vi "初始化检查与创建.vi"(6 "模式(读取)":enum16{"读取", "写入"}(ring), 7 "配置文件 i":T1 {"定时配置-自动导出"."定时配置-自动导出"."间隔" min=1; "定时配置-累积分段"."间隔" min=1}, 8 "error in (no error)":errorcluster caption="错误输入（无错误）", 11 "配置文件路径":path) -> (0 "error out":errorcluster caption="错误输出", 3 "配置文件 o":T1 {"定时配置-自动导出"."定时配置-自动导出"."间隔" min=1; "定时配置-累积分段"."间隔" min=1})   [LabVIEW 2017]
uses:
  a3565fc4-ee2f-4113-b32d-f6e48cc88c0d.vi
  582f122c-475a-4877-9f1d-e028bce6f79a.vi
  9617da62-d855-45df-82b1-57c8dcb712c4.vi
  c94f7198-3dea-4324-b842-01edaf5fdd37.vi
  494809bb-0510-4db4-aacf-66d689d66c07.vi
  <vilib>/Utility/config.llb/Read Key (Boolean).vi
  <vilib>/Utility/config.llb/Write Key (Boolean).vi
  <vilib>/Utility/config.llb/Read Key (String).vi
  <vilib>/Utility/config.llb/Write Key (String).vi
  <vilib>/Utility/config.llb/Read Key (U32).vi
  <vilib>/Utility/config.llb/Write Key (U32).vi
  <vilib>/Utility/config.llb/Write Key (I32).vi
  <vilib>/Utility/config.llb/NI_LVConfig.lvlib
panel:
  in  "键-导出定时配置段":T4
  in  "键-累积定时配置段":T5
  in  "键-串口配置段":T6
  in  "键-杂项段":T7
  in  "段":T8
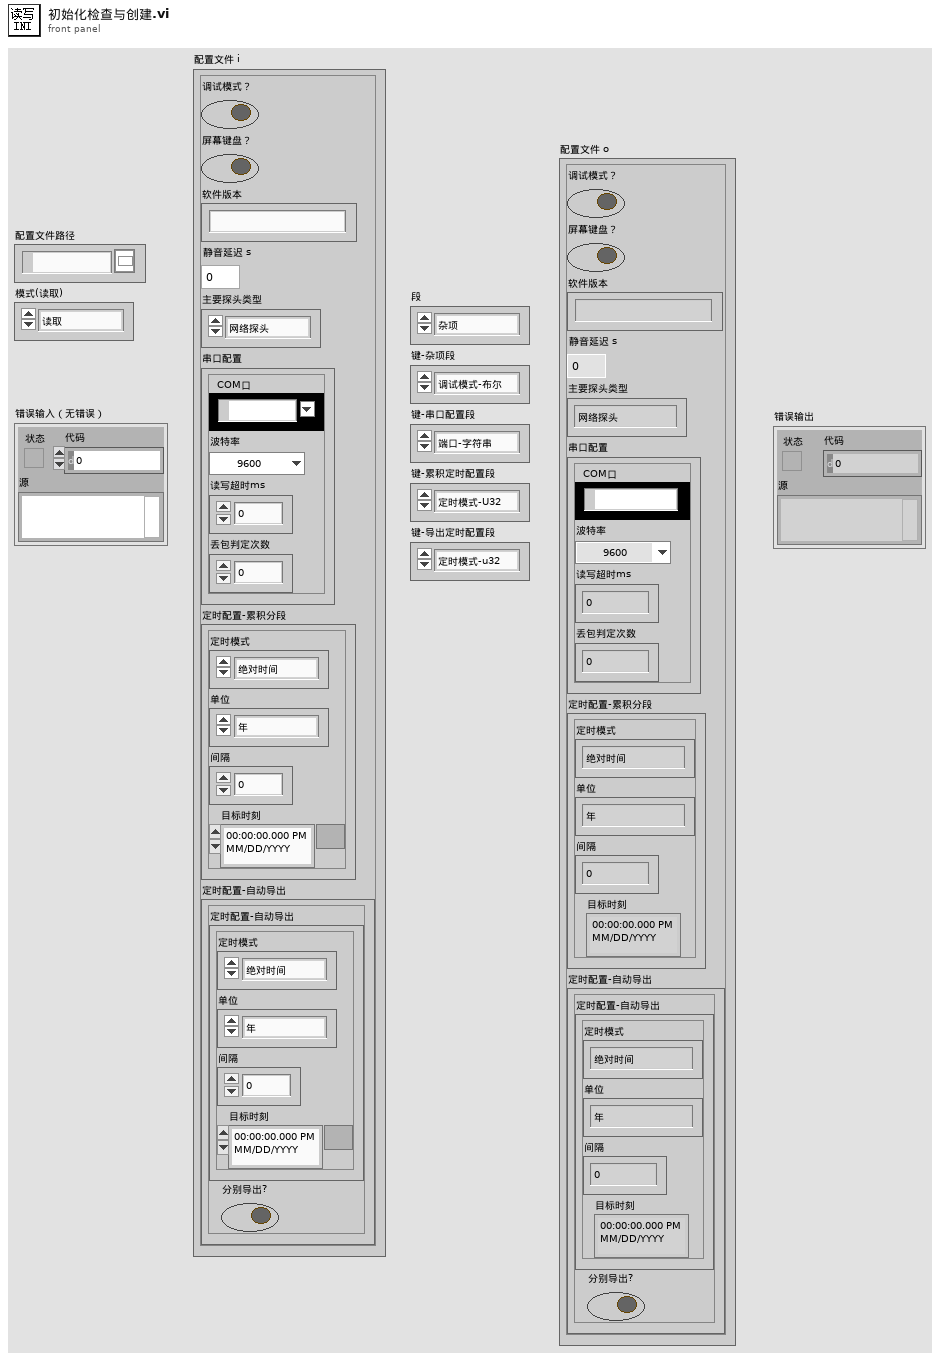
[diagram p1: front panel]
types:
  T1 = typedef "簇-配置文件内容.ctl" = cluster{"调试模式？":bool, "屏幕键盘？":bool, "软件版本":string, "静音延迟 s":u16, "主要探头类型":T2, "串口配置":cluster{"COM口":refnum<visa-resource-name>, "波特率":enum16{"9600", "19200"}, "读写超时ms":i16, "丢包判定次数":i16}, "定时配置-累积分段":T3, "定时配置-自动导出":cluster{"定时配置-自动导出":T3, "分别导出?":bool}}
  T2 = typedef "枚举-主要探头类型.ctl" = enum16{"网络探头", "串口探头"}
  T3 = typedef "簇-定时配置.ctl" = cluster{"定时模式":enum16{"绝对时间", "相对时间"}, "单位":enum16{"年", "月", "日", "时", "分"}, "间隔":u8, "目标时刻":timestamp}
  T4 = typedef "枚举-键-导出定时配置段.ctl" = enum16{"定时模式-u32", "单位-u32", "间隔-u32", "目标时刻-字符串", "分别导出-布尔"}
  T5 = typedef "枚举-键-累积定时配置段.ctl" = enum16{"定时模式-U32", "单位-U32", "间隔-U32", "目标时刻-字符串"}
  T6 = typedef "枚举-键-串口配置段.ctl" = enum16{"端口-字符串", "波特率-U32", "读写超时ms-U32", "丢包判定次数-U32"}
  T7 = typedef "枚举-键-杂项段.ctl" = enum16{"调试模式-布尔", "屏幕键盘-布尔", "软件版本-字符串", "静音延迟-U32", "主要探头类型-U32"}
  T8 = typedef "枚举-段.ctl" = enum16{"杂项", "串口配置", "累积分段定时", "自动导出定时"}
  T9 = cluster{"COM口":refnum<visa-resource-name>, "波特率":enum16{"9600", "19200"}, "读写超时ms":i16, "丢包判定次数":i16}
  T10 = typedef "NI_LVConfig.lvlib/Config Data RefNum.ctl" = refnum<k1>
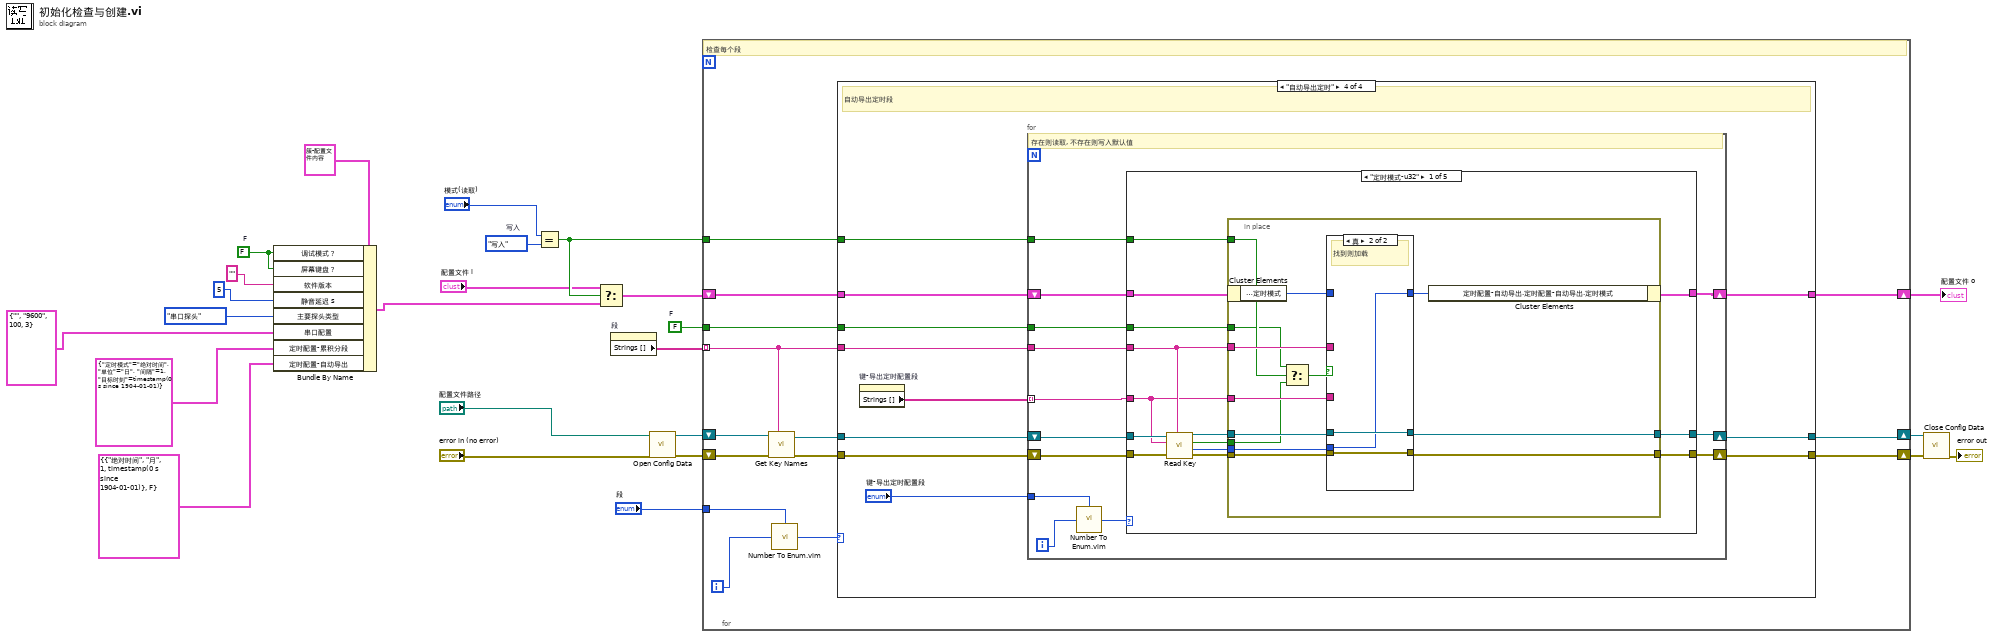
[diagram p0: block diagram]
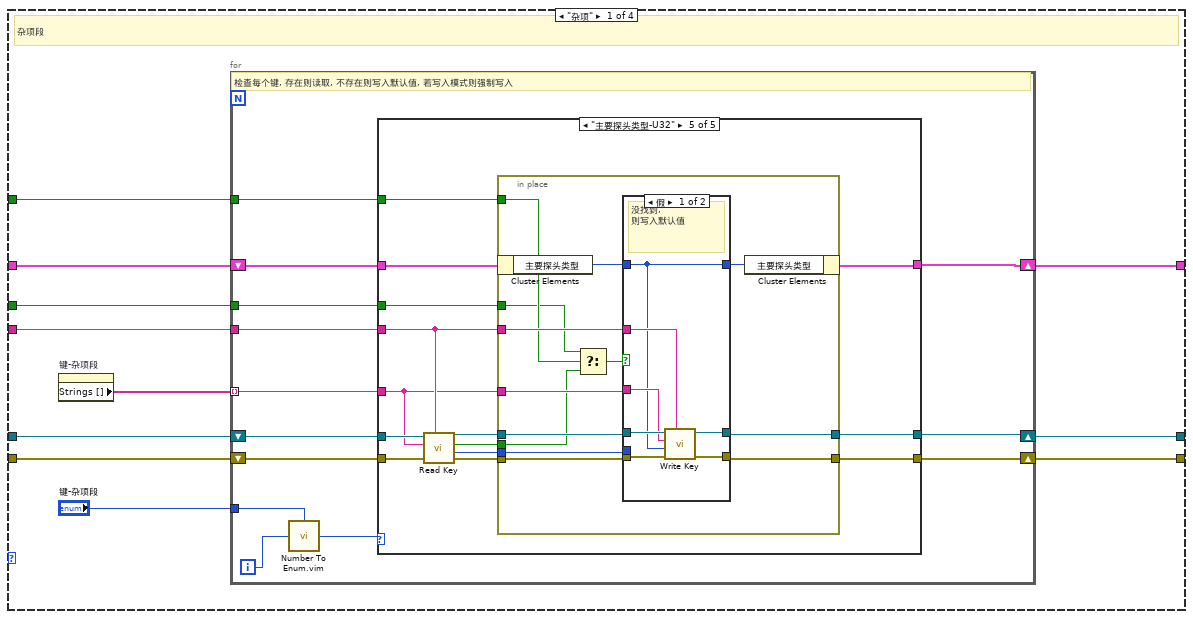
[diagram p2: hidden frame]
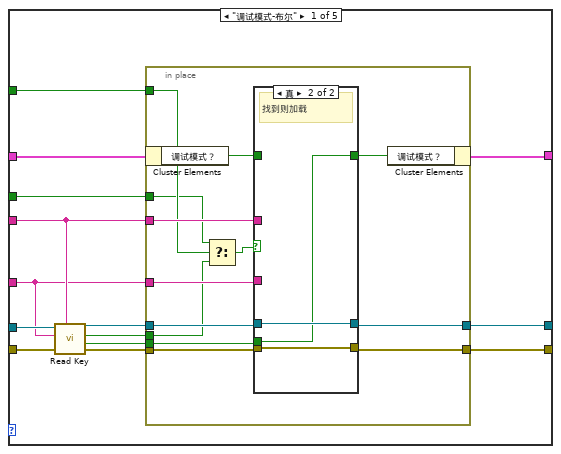
[diagram p3: hidden frame]
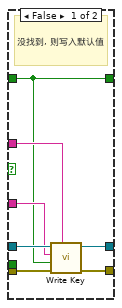
[diagram p4: hidden frame]
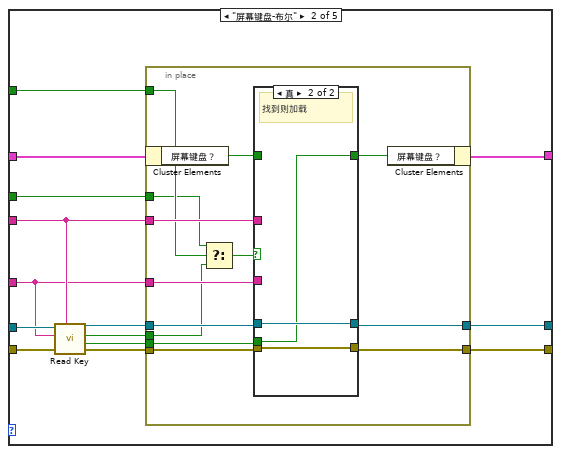
[diagram p5: hidden frame]
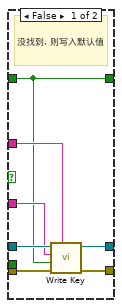
[diagram p6: hidden frame]
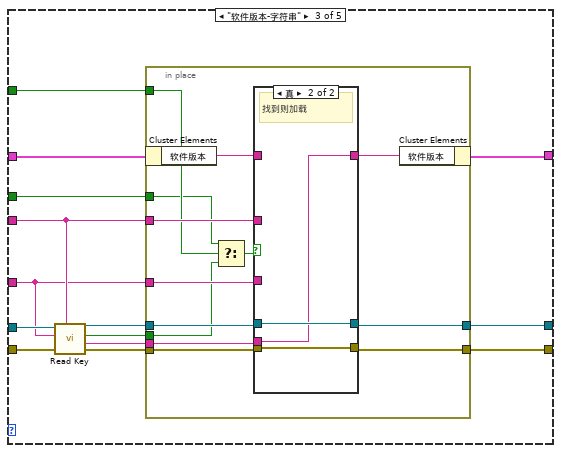
[diagram p7: hidden frame]
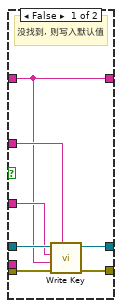
[diagram p8: hidden frame]
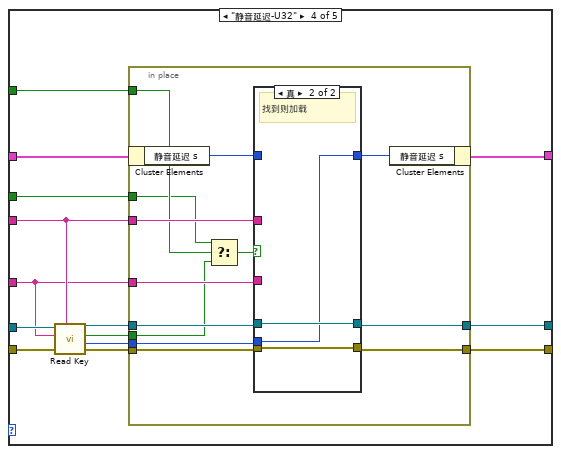
[diagram p9: hidden frame]
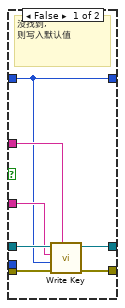
[diagram p10: hidden frame]
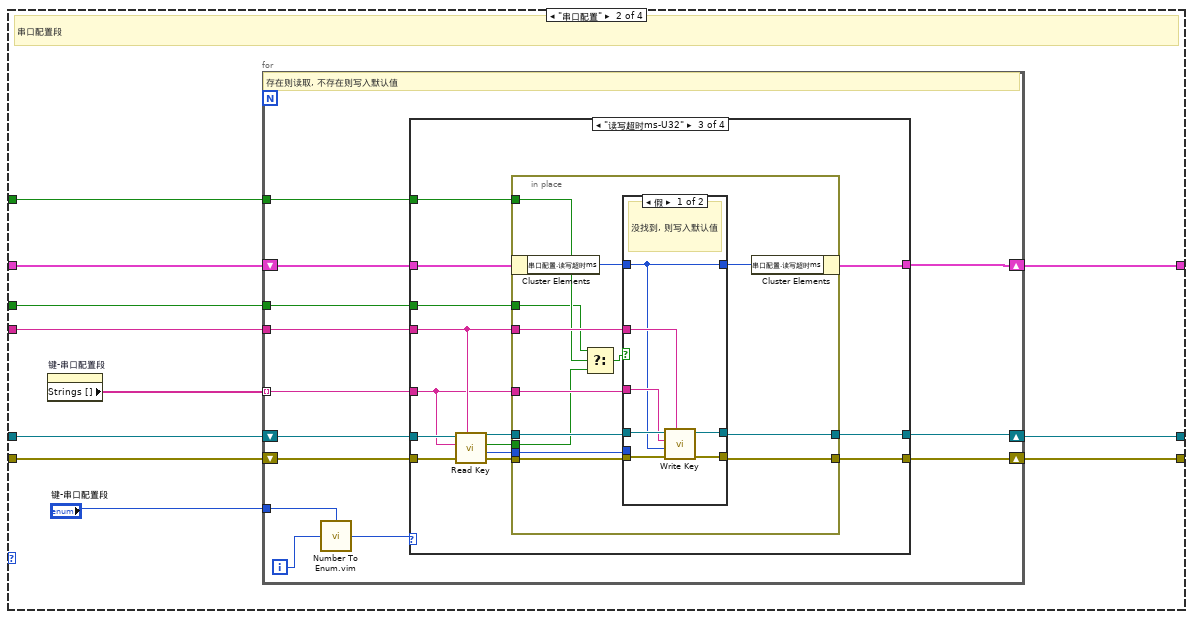
[diagram p12: hidden frame]
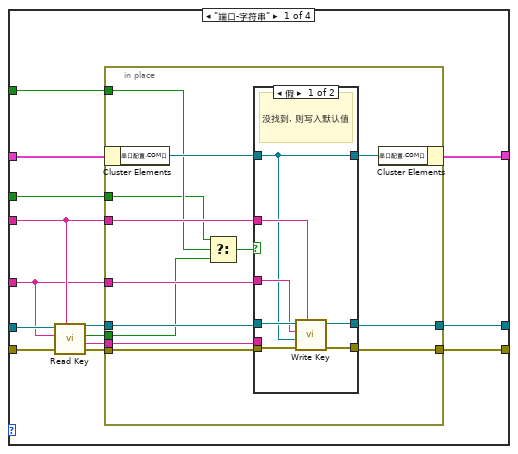
[diagram p13: hidden frame]
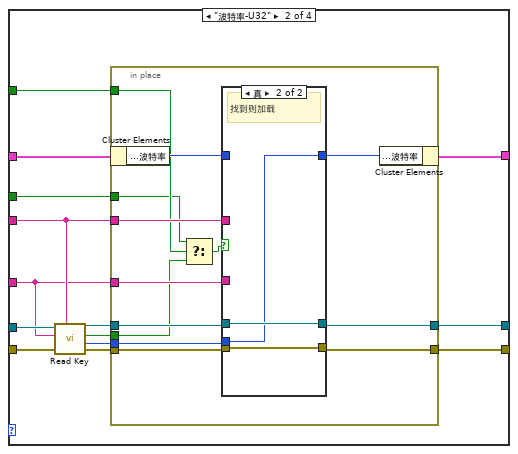
[diagram p15: hidden frame]
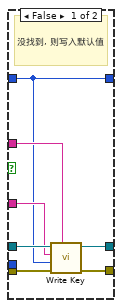
[diagram p16: hidden frame]
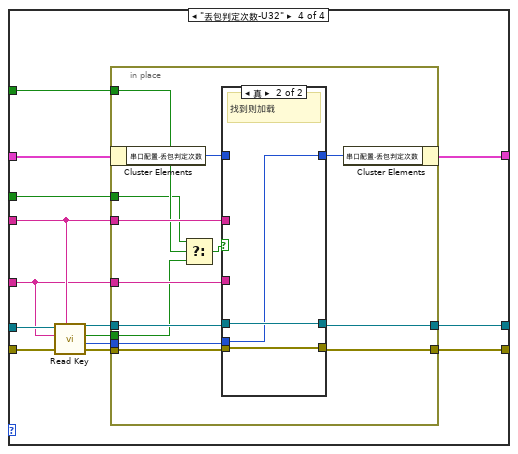
[diagram p18: hidden frame]
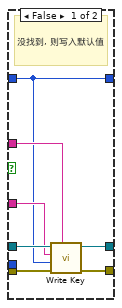
[diagram p19: hidden frame]
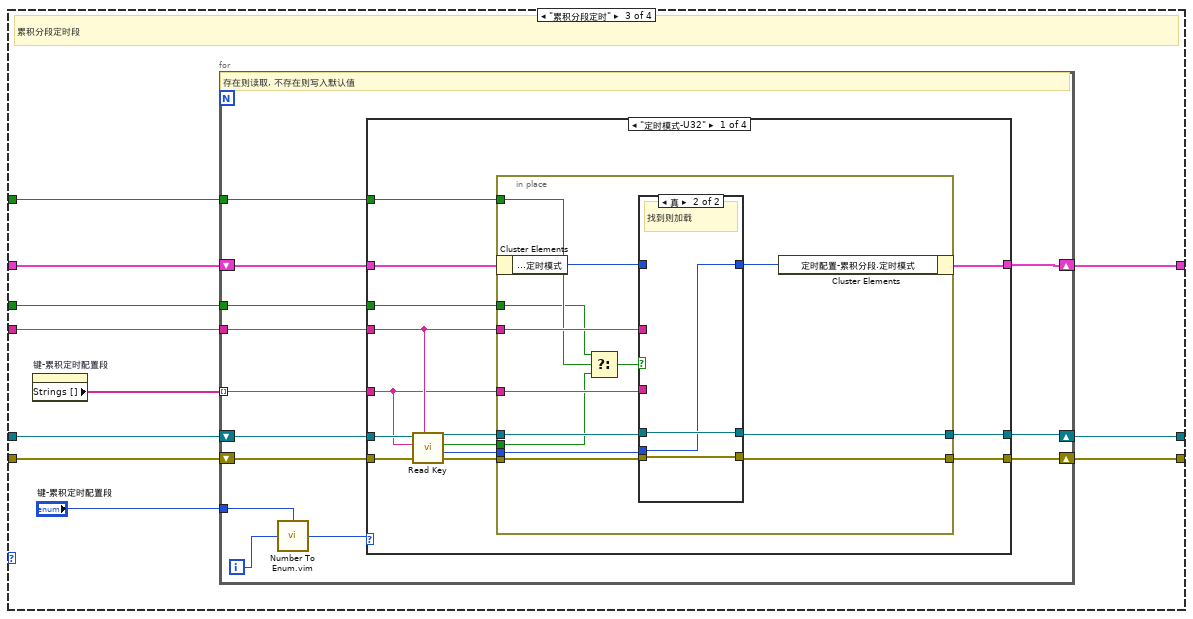
[diagram p20: hidden frame]
diagram:
  w5 = FALSE  # F
  w13 = FALSE  # F
  w14 = enum16{"读取", "写入"}."写入"  # 写入
  n1 = Bundle By Name(cluster=T1 {"调试模式？"=FALSE, "屏幕键盘？"=FALSE, "软件版本"="", "静音延迟 s"=0, "主要探头类型"=enum."网络探头", "串口配置"={"COM口"="", "波特率"=enum."9600", "读写超时ms"=0, "丢包判定次数"=0}, "定时配置-累积分段"={"定时模式"=enum."绝对时间", "单位"=enum."年", "间隔"=0, "目标时刻"=timestamp(0 s since 1904-01-01)}, "定时配置-自动导出"={"定时配置-自动导出"={"定时模式"=enum."绝对时间", "单位"=enum."年", "间隔"=0, "目标时刻"=timestamp(0 s since 1904-01-01)}, "分别导出?"=FALSE}} ("配置文件 i"), "调试模式？"=w5, "屏幕键盘？"=w5, "软件版本"="", "静音延迟 s"=u16 5, "主要探头类型"=枚举-主要探头类型."串口探头", "串口配置"=T9 {"COM口"="", "波特率"=enum."9600", "读写超时ms"=100, "丢包判定次数"=3}, "定时配置-累积分段"=T3 {"定时模式"=enum."绝对时间", "单位"=enum."日", "间隔"=1, "目标时刻"=timestamp(0 s since 1904-01-01)}, "定时配置-自动导出"=cluster{"定时配置-自动导出":T3, "分别导出?":bool} {"定时配置-自动导出"={"定时模式"=enum."绝对时间", "单位"=enum."月", "间隔"=1, "目标时刻"=timestamp(0 s since 1904-01-01)}, "分别导出?"=FALSE}) -> (w3:T1)
  n2 = Equal?(x="模式(读取)", y=w14) -> (x = y?=w12:bool)
  n3 = Select(t="配置文件 i", s=w12, f=w3) -> (s? t:f=w10:T1)
  n4 = property on="段" class="Enum (严格)"() -> ("Strings []"=w23:string[])  [unwired: 2 in, 2 out]
  n5 = call <vilib>:"Open Config Data.vi"("error in (no error)"="error in (no error)", "configuration file path"="配置文件路径") -> ("error out"=w17:errorcluster, "refnum"=w24:T10)  [unwired: 7 in, 1 out]
  n6 = for {
    tunnel: w23 -> [w34] mode=indexing
    shift-right: [w28] -> w22
    shift-left: w10 -> [w33]
    shift-right: [w29] -> w19
    shift-left: w24 -> [w39]
    shift-right: [w30] -> w20
    shift-left: w17 -> [w31]
    tunnel: "段" -> [w36]
    tunnel: w12 -> [w27]
    tunnel: w13 -> [w26]
    i -> [w37]
    # "检查每个段"
    n7 = call <vilib>:"Get Key Names.vi"("section"=w34, "error in (no error)"=w31, "refnum"=w39) -> ("error out"=w32:errorcluster, "refnum out"=w38:T10)  [unwired: 5 in, 2 out]
    n8 = call "Number To Enum.vim"("number"=w37, "enum type"=w36) -> ("number as enum"=w35:T8)
    n9 = case shown="\"自动导出定时\"" w35 {
      tunnel: w38 -> [w49 w259 w431 w606]
      tunnel: w34 -> [w48 w258 w430 w605]
      tunnel: w33 -> [w47 w257 w429 w604]
      tunnel: w32 -> [w45 w256 w428 w603]
      tunnel: [w44 w255 w427 w602] -> w30
      tunnel: [w43 w254 w426 w601] -> w29
      tunnel: [w42 w251 w423 w598] -> w28
      tunnel: w27 -> [w41 w250 w421 w597]
      tunnel: w26 -> [w40 w249 w422 w596]
      frame "杂项" {
        # "杂项段"
        n10 = property on="键-杂项段" class="Enum (严格)"() -> ("Strings []"=w50:string[])  [unwired: 2 in, 2 out]
        n11 = for {
          tunnel: w50 -> [w61] mode=indexing
          tunnel: w48 -> [w62]
          shift-right: [w53] -> w42
          shift-left: w47 -> [w57]
          tunnel: "键-杂项段" -> [w59]
          shift-right: [w54] -> w43
          shift-left: w49 -> [w63]
          shift-right: [w55] -> w44
          shift-left: w45 -> [w56]
          tunnel: w41 -> [w52]
          tunnel: w40 -> [w51]
          i -> [w60]
          # "检查每个键, 存在则读取, 不存在则写入默认值, 若写入模式则强制写入"
          n12 = call "Number To Enum.vim"("number"=w60, "enum type"=w59) -> ("number as enum"=w58:T7)
          n13 = case shown="\"主要探头类型-U32\"" w58 {
            tunnel: w63 -> [w77 w114 w151 w188 w225]
            tunnel: w62 -> [w74 w111 w148 w185 w222]
            tunnel: w61 -> [w73 w110 w147 w184 w221]
            tunnel: w57 -> [w67 w104 w141 w178 w215]
            tunnel: w56 -> [w71 w108 w145 w182 w219]
            tunnel: [w70 w107 w144 w181 w218] -> w55
            tunnel: [w69 w106 w143 w180 w217] -> w54
            tunnel: [w66 w103 w140 w177 w214] -> w53
            tunnel: w52 -> [w65 w102 w139 w176 w213]
            tunnel: w51 -> [w64 w101 w138 w175 w212]
            frame "调试模式-布尔" {
              n14 = call-poly <vilib>:"Read Key.vi"("section"=w74, "error in (no error)"=w71, "key"=w73, "refnum"=w77) -> ("error out"=w72:errorcluster, "value"=w68:bool, "found?"=w76:bool, "refnum out"=w75:T10)  [unwired: 4 in]
              n15 = in-place {
                in-place-border: w76 -> [w79]
                in-place-border: w75 -> [w90]
                in-place-border: w74 -> [w89]
                in-place-border: w73 -> [w88]
                in-place-border: w72 -> [w87]
                in-place-border: [w86] -> w70
                in-place-border: [w85] -> w69
                in-place-border: w68 -> [w84]
                in-place-border: w65 -> [w81]
                in-place-border: w64 -> [w80]
                n16 = in-place-cluster #1(w67) -> ("调试模式？"=w82:bool)
                n17 = Select(t=w80, s=w81, f=w79) -> (s? t:f=w78:bool)
                n18 = case shown="真" w78 {
                  tunnel: w90 -> [w97 w99]
                  tunnel: w89 -> [w96 _]
                  tunnel: w88 -> [w95 _]
                  tunnel: w87 -> [w94 w100]
                  tunnel: [w93 w100] -> w86
                  tunnel: [w92 w99] -> w85
                  tunnel: w84 -> [_ w98]
                  tunnel: [w91 w98] -> w83
                  tunnel: w82 -> [w91 _]
                  frame False {
                    # "没找到, 则写入默认值"
                    n19 = call-poly <vilib>:"Write Key.vi"("section"=w96, "error in (no error)"=w94, "value"=w91, "key"=w95, "refnum"=w97) -> ("error out"=w93:errorcluster, "refnum out"=w92:T10)  [unwired: 4 in, 1 out]
                  }
                  frame True {
                    # "找到则加载"
                  }
                }
                n20 = in-place-cluster #1("调试模式？"=w83) -> (w66:T1)
              }
            }
            frame "屏幕键盘-布尔" {
              n21 = call-poly <vilib>:"Read Key.vi"("section"=w111, "error in (no error)"=w108, "key"=w110, "refnum"=w114) -> ("error out"=w109:errorcluster, "value"=w105:bool, "found?"=w113:bool, "refnum out"=w112:T10)  [unwired: 4 in]
              n22 = in-place {
                in-place-border: w113 -> [w116]
                in-place-border: w112 -> [w127]
                in-place-border: w111 -> [w126]
                in-place-border: w110 -> [w125]
                in-place-border: w109 -> [w124]
                in-place-border: [w123] -> w107
                in-place-border: [w122] -> w106
                in-place-border: w105 -> [w121]
                in-place-border: w102 -> [w118]
                in-place-border: w101 -> [w117]
                n23 = in-place-cluster #2(w104) -> ("屏幕键盘？"=w119:bool)
                n24 = Select(t=w117, s=w118, f=w116) -> (s? t:f=w115:bool)
                n25 = case shown="真" w115 {
                  tunnel: w127 -> [w134 w136]
                  tunnel: w126 -> [w133 _]
                  tunnel: w125 -> [w132 _]
                  tunnel: w124 -> [w131 w137]
                  tunnel: [w130 w137] -> w123
                  tunnel: [w129 w136] -> w122
                  tunnel: w121 -> [_ w135]
                  tunnel: [w128 w135] -> w120
                  tunnel: w119 -> [w128 _]
                  frame False {
                    # "没找到, 则写入默认值"
                    n26 = call-poly <vilib>:"Write Key.vi"("section"=w133, "error in (no error)"=w131, "value"=w128, "key"=w132, "refnum"=w134) -> ("error out"=w130:errorcluster, "refnum out"=w129:T10)  [unwired: 4 in, 1 out]
                  }
                  frame True {
                    # "找到则加载"
                  }
                }
                n27 = in-place-cluster #2("屏幕键盘？"=w120) -> (w103:T1)
              }
            }
            frame "软件版本-字符串" {
              n28 = call-poly <vilib>:"Read Key.vi"("section"=w148, "error in (no error)"=w145, "key"=w147, "refnum"=w151) -> ("error out"=w146:errorcluster, "value"=w142:string, "found?"=w150:bool, "refnum out"=w149:T10)  [unwired: 4 in]
              n29 = in-place {
                in-place-border: w150 -> [w153]
                in-place-border: w149 -> [w164]
                in-place-border: w148 -> [w163]
                in-place-border: w147 -> [w162]
                in-place-border: w146 -> [w161]
                in-place-border: [w160] -> w144
                in-place-border: [w159] -> w143
                in-place-border: w142 -> [w158]
                in-place-border: w139 -> [w155]
                in-place-border: w138 -> [w154]
                n30 = in-place-cluster #3(w141) -> ("软件版本"=w156:string)
                n31 = Select(t=w154, s=w155, f=w153) -> (s? t:f=w152:bool)
                n32 = case shown="真" w152 {
                  tunnel: w164 -> [w171 w173]
                  tunnel: w163 -> [w170 _]
                  tunnel: w162 -> [w169 _]
                  tunnel: w161 -> [w168 w174]
                  tunnel: [w167 w174] -> w160
                  tunnel: [w166 w173] -> w159
                  tunnel: w158 -> [_ w172]
                  tunnel: [w165 w172] -> w157
                  tunnel: w156 -> [w165 _]
                  frame False {
                    # "没找到, 则写入默认值"
                    n33 = call-poly <vilib>:"Write Key.vi"("section"=w170, "error in (no error)"=w168, "value"=w165, "key"=w169, "refnum"=w171) -> ("error out"=w167:errorcluster, "refnum out"=w166:T10)  [unwired: 4 in, 1 out]
                  }
                  frame True {
                    # "找到则加载"
                  }
                }
                n34 = in-place-cluster #3("软件版本"=w157) -> (w140:T1)
              }
            }
            frame "静音延迟-U32" {
              n35 = call-poly <vilib>:"Read Key.vi"("section"=w185, "error in (no error)"=w182, "key"=w184, "refnum"=w188) -> ("error out"=w183:errorcluster, "value"=w179:u32, "found?"=w187:bool, "refnum out"=w186:T10)  [unwired: 4 in]
              n36 = in-place {
                in-place-border: w187 -> [w190]
                in-place-border: w186 -> [w201]
                in-place-border: w185 -> [w200]
                in-place-border: w184 -> [w199]
                in-place-border: w183 -> [w198]
                in-place-border: [w197] -> w181
                in-place-border: [w196] -> w180
                in-place-border: w179 -> [w195]
                in-place-border: w176 -> [w192]
                in-place-border: w175 -> [w191]
                n37 = in-place-cluster #4(w178) -> ("静音延迟 s"=w193:u16)
                n38 = Select(t=w191, s=w192, f=w190) -> (s? t:f=w189:bool)
                n39 = case shown="真" w189 {
                  tunnel: w201 -> [w208 w210]
                  tunnel: w200 -> [w207 _]
                  tunnel: w199 -> [w206 _]
                  tunnel: w198 -> [w205 w211]
                  tunnel: [w204 w211] -> w197
                  tunnel: [w203 w210] -> w196
                  tunnel: w195 -> [_ w209]
                  tunnel: [w202 w209] -> w194
                  tunnel: w193 -> [w202 _]
                  frame False {
                    # "没找到, \n则写入默认值"
                    n40 = call-poly <vilib>:"Write Key.vi"("section"=w207, "error in (no error)"=w205, "value"=w202, "key"=w206, "refnum"=w208) -> ("error out"=w204:errorcluster, "refnum out"=w203:T10)  [unwired: 4 in, 1 out]
                  }
                  frame True {
                    # "找到则加载"
                  }
                }
                n41 = in-place-cluster #4("静音延迟 s"=w194) -> (w177:T1)
              }
            }
            frame "主要探头类型-U32" {
              n42 = call-poly <vilib>:"Read Key.vi"("section"=w222, "error in (no error)"=w219, "key"=w221, "refnum"=w225) -> ("error out"=w220:errorcluster, "value"=w216:u32, "found?"=w224:bool, "refnum out"=w223:T10)  [unwired: 4 in]
              n43 = in-place {
                in-place-border: w224 -> [w227]
                in-place-border: w223 -> [w238]
                in-place-border: w222 -> [w237]
                in-place-border: w221 -> [w236]
                in-place-border: w220 -> [w235]
                in-place-border: [w234] -> w218
                in-place-border: [w233] -> w217
                in-place-border: w216 -> [w232]
                in-place-border: w213 -> [w229]
                in-place-border: w212 -> [w228]
                n44 = in-place-cluster #5(w215) -> ("主要探头类型"=w230:T2)
                n45 = Select(t=w228, s=w229, f=w227) -> (s? t:f=w226:bool)
                n46 = case shown="假" w226 {
                  tunnel: w238 -> [w245 w247]
                  tunnel: w237 -> [w244 _]
                  tunnel: w236 -> [w243 _]
                  tunnel: w235 -> [w242 w248]
                  tunnel: [w241 w248] -> w234
                  tunnel: [w240 w247] -> w233
                  tunnel: w232 -> [_ w246]
                  tunnel: [w239 w246] -> w231
                  tunnel: w230 -> [w239 _]
                  frame False {
                    # "没找到, \n则写入默认值"
                    n47 = call-poly <vilib>:"Write Key.vi"("section"=w244, "error in (no error)"=w242, "value"=w239, "key"=w243, "refnum"=w245) -> ("error out"=w241:errorcluster, "refnum out"=w240:T10)  [unwired: 4 in, 1 out]
                  }
                  frame True {
                    # "找到则加载"
                  }
                }
                n48 = in-place-cluster #5("主要探头类型"=w231) -> (w214:T1)
              }
            }
          }
        }
      }
      frame "串口配置" {
        # "串口配置段"
        n49 = property on="键-串口配置段" class="Enum (严格)"() -> ("Strings []"=w252:string[])  [unwired: 2 in, 2 out]
        n50 = for {
          tunnel: w252 -> [w270] mode=indexing
          tunnel: w258 -> [w271]
          shift-right: [w262] -> w251
          shift-left: w257 -> [w266]
          tunnel: "键-串口配置段" -> [w268]
          shift-right: [w263] -> w254
          shift-left: w259 -> [w272]
          shift-right: [w264] -> w255
          shift-left: w256 -> [w265]
          tunnel: w250 -> [w261]
          tunnel: w249 -> [w260]
          i -> [w269]
          # "存在则读取, 不存在则写入默认值"
          n51 = call "Number To Enum.vim"("number"=w269, "enum type"=w268) -> ("number as enum"=w267:T6)
          n52 = case shown="\"读写超时ms-U32\"" w267 {
            tunnel: w272 -> [w286 w323 w360 w397]
            tunnel: w271 -> [w283 w320 w357 w394]
            tunnel: w270 -> [w282 w319 w356 w393]
            tunnel: w266 -> [w276 w313 w350 w387]
            tunnel: w265 -> [w280 w317 w354 w391]
            tunnel: [w279 w316 w353 w390] -> w264
            tunnel: [w278 w315 w352 w389] -> w263
            tunnel: [w275 w312 w349 w386] -> w262
            tunnel: w261 -> [w274 w311 w348 w385]
            tunnel: w260 -> [w273 w310 w347 w384]
            frame "端口-字符串" {
              n53 = call-poly <vilib>:"Read Key.vi"("section"=w283, "error in (no error)"=w280, "key"=w282, "refnum"=w286) -> ("error out"=w281:errorcluster, "value"=w277:string, "found?"=w285:bool, "refnum out"=w284:T10)  [unwired: 4 in]
              n54 = in-place {
                in-place-border: w285 -> [w288]
                in-place-border: w284 -> [w299]
                in-place-border: w283 -> [w298]
                in-place-border: w282 -> [w297]
                in-place-border: w281 -> [w296]
                in-place-border: [w295] -> w279
                in-place-border: [w294] -> w278
                in-place-border: w277 -> [w293]
                in-place-border: w274 -> [w290]
                in-place-border: w273 -> [w289]
                n55 = in-place-cluster #6(w276) -> ("串口配置.COM口"=w291:refnum<visa-resource-name>)
                n56 = Select(t=w289, s=w290, f=w288) -> (s? t:f=w287:bool)
                n57 = case shown="假" w287 {
                  tunnel: w299 -> [w306 w308]
                  tunnel: w298 -> [w305 _]
                  tunnel: w297 -> [w304 _]
                  tunnel: w296 -> [w303 w309]
                  tunnel: [w302 w309] -> w295
                  tunnel: [w301 w308] -> w294
                  tunnel: w293 -> [_ w307]
                  tunnel: [w300 w307] -> w292
                  tunnel: w291 -> [w300 _]
                  frame False {
                    # "没找到, 则写入默认值"
                    n58 = call-poly <vilib>:"Write Key.vi"("section"=w305, "error in (no error)"=w303, "value"=w300, "key"=w304, "refnum"=w306) -> ("error out"=w302:errorcluster, "refnum out"=w301:T10)  [unwired: 4 in, 1 out]
                  }
                  frame True {
                    # "找到则加载"
                  }
                }
                n59 = in-place-cluster #6("串口配置.COM口"=w292) -> (w275:T1)
              }
            }
            frame "波特率-U32" {
              n60 = call-poly <vilib>:"Read Key.vi"("section"=w320, "error in (no error)"=w317, "key"=w319, "refnum"=w323) -> ("error out"=w318:errorcluster, "value"=w314:u32, "found?"=w322:bool, "refnum out"=w321:T10)  [unwired: 4 in]
              n61 = in-place {
                in-place-border: w322 -> [w325]
                in-place-border: w321 -> [w336]
                in-place-border: w320 -> [w335]
                in-place-border: w319 -> [w334]
                in-place-border: w318 -> [w333]
                in-place-border: [w332] -> w316
                in-place-border: [w331] -> w315
                in-place-border: w314 -> [w330]
                in-place-border: w311 -> [w327]
                in-place-border: w310 -> [w326]
                n62 = in-place-cluster #7(w313) -> ("串口配置.波特率"=w328:enum16{"9600", "19200"})
                n63 = Select(t=w326, s=w327, f=w325) -> (s? t:f=w324:bool)
                n64 = case shown="真" w324 {
                  tunnel: w336 -> [w343 w345]
                  tunnel: w335 -> [w342 _]
                  tunnel: w334 -> [w341 _]
                  tunnel: w333 -> [w340 w346]
                  tunnel: [w339 w346] -> w332
                  tunnel: [w338 w345] -> w331
                  tunnel: w330 -> [_ w344]
                  tunnel: [w337 w344] -> w329
                  tunnel: w328 -> [w337 _]
                  frame False {
                    # "没找到, 则写入默认值"
                    n65 = call-poly <vilib>:"Write Key.vi"("section"=w342, "error in (no error)"=w340, "value"=w337, "key"=w341, "refnum"=w343) -> ("error out"=w339:errorcluster, "refnum out"=w338:T10)  [unwired: 4 in, 1 out]
                  }
                  frame True {
                    # "找到则加载"
                  }
                }
                n66 = in-place-cluster #7("串口配置.波特率"=w329) -> (w312:T1)
              }
            }
            frame "读写超时ms-U32" {
              n67 = call-poly <vilib>:"Read Key.vi"("section"=w357, "error in (no error)"=w354, "key"=w356, "refnum"=w360) -> ("error out"=w355:errorcluster, "value"=w351:u32, "found?"=w359:bool, "refnum out"=w358:T10)  [unwired: 4 in]
              n68 = in-place {
                in-place-border: w359 -> [w362]
                in-place-border: w358 -> [w373]
                in-place-border: w357 -> [w372]
                in-place-border: w356 -> [w371]
                in-place-border: w355 -> [w370]
                in-place-border: [w369] -> w353
                in-place-border: [w368] -> w352
                in-place-border: w351 -> [w367]
                in-place-border: w348 -> [w364]
                in-place-border: w347 -> [w363]
                n69 = in-place-cluster #8(w350) -> ("串口配置.读写超时ms"=w365:i16)
                n70 = Select(t=w363, s=w364, f=w362) -> (s? t:f=w361:bool)
                n71 = case shown="假" w361 {
                  tunnel: w373 -> [w380 w382]
                  tunnel: w372 -> [w379 _]
                  tunnel: w371 -> [w378 _]
                  tunnel: w370 -> [w377 w383]
                  tunnel: [w376 w383] -> w369
                  tunnel: [w375 w382] -> w368
                  tunnel: w367 -> [_ w381]
                  tunnel: [w374 w381] -> w366
                  tunnel: w365 -> [w374 _]
                  frame False {
                    # "没找到, 则写入默认值"
                    n72 = call-poly <vilib>:"Write Key.vi"("section"=w379, "error in (no error)"=w377, "value"=w374, "key"=w378, "refnum"=w380) -> ("error out"=w376:errorcluster, "refnum out"=w375:T10)  [unwired: 4 in, 1 out]
                  }
                  frame True {
                    # "找到则加载"
                  }
                }
                n73 = in-place-cluster #8("串口配置.读写超时ms"=w366) -> (w349:T1)
              }
            }
            frame "丢包判定次数-U32" {
              n74 = call-poly <vilib>:"Read Key.vi"("section"=w394, "error in (no error)"=w391, "key"=w393, "refnum"=w397) -> ("error out"=w392:errorcluster, "value"=w388:u32, "found?"=w396:bool, "refnum out"=w395:T10)  [unwired: 4 in]
              n75 = in-place {
                in-place-border: w396 -> [w399]
                in-place-border: w395 -> [w410]
                in-place-border: w394 -> [w409]
                in-place-border: w393 -> [w408]
                in-place-border: w392 -> [w407]
                in-place-border: [w406] -> w390
                in-place-border: [w405] -> w389
                in-place-border: w388 -> [w404]
                in-place-border: w385 -> [w401]
                in-place-border: w384 -> [w400]
                n76 = in-place-cluster #9(w387) -> ("串口配置.丢包判定次数"=w402:i16)
                n77 = Select(t=w400, s=w401, f=w399) -> (s? t:f=w398:bool)
                n78 = case shown="真" w398 {
                  tunnel: w410 -> [w417 w419]
                  tunnel: w409 -> [w416 _]
                  tunnel: w408 -> [w415 _]
                  tunnel: w407 -> [w414 w420]
                  tunnel: [w413 w420] -> w406
                  tunnel: [w412 w419] -> w405
                  tunnel: w404 -> [_ w418]
                  tunnel: [w411 w418] -> w403
                  tunnel: w402 -> [w411 _]
                  frame False {
                    # "没找到, 则写入默认值"
                    n79 = call-poly <vilib>:"Write Key.vi"("section"=w416, "error in (no error)"=w414, "value"=w411, "key"=w415, "refnum"=w417) -> ("error out"=w413:errorcluster, "refnum out"=w412:T10)  [unwired: 4 in, 1 out]
                  }
                  frame True {
                    # "找到则加载"
                  }
                }
                n80 = in-place-cluster #9("串口配置.丢包判定次数"=w403) -> (w386:T1)
              }
            }
          }
        }
      }
      frame "累积分段定时" {
        # "累积分段定时段"
        n81 = property on="键-累积定时配置段" class="Enum (严格)"() -> ("Strings []"=w424:string[])  [unwired: 2 in, 2 out]
        n82 = for {
          tunnel: w424 -> [w442] mode=indexing
          tunnel: w430 -> [w443]
          shift-right: [w434] -> w423
          shift-left: w429 -> [w438]
          tunnel: "键-累积定时配置段" -> [w440]
          shift-right: [w435] -> w426
          shift-left: w431 -> [w444]
          shift-right: [w436] -> w427
          shift-left: w428 -> [w437]
          tunnel: w422 -> [w433]
          tunnel: w421 -> [w432]
          i -> [w441]
          # "存在则读取, 不存在则写入默认值"
          n83 = call "Number To Enum.vim"("number"=w441, "enum type"=w440) -> ("number as enum"=w439:T5)
          n84 = case shown="\"定时模式-U32\"" w439 {
            tunnel: w444 -> [w458 w495 w532 w569]
            tunnel: w443 -> [w455 w492 w529 w566]
            tunnel: w442 -> [w454 w491 w528 w565]
            tunnel: w438 -> [w448 w485 w522 w559]
            tunnel: w437 -> [w452 w489 w526 w563]
            tunnel: [w451 w488 w525 w562] -> w436
            tunnel: [w450 w487 w524 w561] -> w435
            tunnel: [w447 w484 w521 w558] -> w434
            tunnel: w433 -> [w445 w482 w519 w557]
            tunnel: w432 -> [w446 w483 w520 w556]
            frame "定时模式-U32" {
              n85 = call-poly <vilib>:"Read Key.vi"("section"=w455, "error in (no error)"=w452, "key"=w454, "refnum"=w458) -> ("error out"=w453:errorcluster, "value"=w449:u32, "found?"=w457:bool, "refnum out"=w456:T10)  [unwired: 4 in]
              n86 = in-place {
                in-place-border: w457 -> [w460]
                in-place-border: w456 -> [w471]
                in-place-border: w455 -> [w470]
                in-place-border: w454 -> [w469]
                in-place-border: w453 -> [w468]
                in-place-border: [w467] -> w451
                in-place-border: [w466] -> w450
                in-place-border: w449 -> [w465]
                in-place-border: w446 -> [w462]
                in-place-border: w445 -> [w461]
                n87 = in-place-cluster #10(w448) -> ("定时配置-累积分段.定时模式"=w463:enum16{"绝对时间", "相对时间"})
                n88 = Select(t=w461, s=w462, f=w460) -> (s? t:f=w459:bool)
                n89 = case shown="真" w459 {
                  tunnel: w471 -> [w478 w480]
                  tunnel: w470 -> [w477 _]
                  tunnel: w469 -> [w476 _]
                  tunnel: w468 -> [w475 w481]
                  tunnel: [w474 w481] -> w467
                  tunnel: [w473 w480] -> w466
                  tunnel: w465 -> [_ w479]
                  tunnel: [w472 w479] -> w464
                  tunnel: w463 -> [w472 _]
                  frame False {
                    # "没找到, 则写入默认值"
                    n90 = call-poly <vilib>:"Write Key.vi"("section"=w477, "error in (no error)"=w475, "value"=w472, "key"=w476, "refnum"=w478) -> ("error out"=w474:errorcluster, "refnum out"=w473:T10)  [unwired: 4 in, 1 out]
                  }
                  frame True {
                    # "找到则加载"
                  }
                }
                n91 = in-place-cluster #10("定时配置-累积分段.定时模式"=w464) -> (w447:T1)
              }
            }
            frame "单位-U32" {
              n92 = call-poly <vilib>:"Read Key.vi"("section"=w492, "error in (no error)"=w489, "key"=w491, "refnum"=w495) -> ("error out"=w490:errorcluster, "value"=w486:u32, "found?"=w494:bool, "refnum out"=w493:T10)  [unwired: 4 in]
              n93 = in-place {
                in-place-border: w494 -> [w497]
                in-place-border: w493 -> [w508]
                in-place-border: w492 -> [w507]
                in-place-border: w491 -> [w506]
                in-place-border: w490 -> [w505]
                in-place-border: [w504] -> w488
                in-place-border: [w503] -> w487
                in-place-border: w486 -> [w502]
                in-place-border: w483 -> [w499]
                in-place-border: w482 -> [w498]
                n94 = in-place-cluster #11(w485) -> ("定时配置-累积分段.单位"=w500:enum16{"年", "月", "日", "时", "分"})
                n95 = Select(t=w498, s=w499, f=w497) -> (s? t:f=w496:bool)
                n96 = case shown="真" w496 {
                  tunnel: w508 -> [w515 w517]
                  tunnel: w507 -> [w514 _]
                  tunnel: w506 -> [w513 _]
                  tunnel: w505 -> [w512 w518]
                  tunnel: [w511 w518] -> w504
                  tunnel: [w510 w517] -> w503
                  tunnel: w502 -> [_ w516]
                  tunnel: [w509 w516] -> w501
                  tunnel: w500 -> [w509 _]
                  frame False {
                    # "没找到, 则写入默认值"
                    n97 = call-poly <vilib>:"Write Key.vi"("section"=w514, "error in (no error)"=w512, "value"=w509, "key"=w513, "refnum"=w515) -> ("error out"=w511:errorcluster, "refnum out"=w510:T10)  [unwired: 4 in, 1 out]
                  }
                  frame True {
                    # "找到则加载"
                  }
                }
                n98 = in-place-cluster #11("定时配置-累积分段.单位"=w501) -> (w484:T1)
              }
            }
            frame "间隔-U32" {
              n99 = call-poly <vilib>:"Read Key.vi"("section"=w529, "error in (no error)"=w526, "key"=w528, "refnum"=w532) -> ("error out"=w527:errorcluster, "value"=w523:u32, "found?"=w531:bool, "refnum out"=w530:T10)  [unwired: 4 in]
              n100 = in-place {
                in-place-border: w531 -> [w534]
                in-place-border: w530 -> [w545]
                in-place-border: w529 -> [w544]
                in-place-border: w528 -> [w543]
                in-place-border: w527 -> [w542]
                in-place-border: [w541] -> w525
                in-place-border: [w540] -> w524
                in-place-border: w523 -> [w539]
                in-place-border: w520 -> [w536]
                in-place-border: w519 -> [w535]
                n101 = in-place-cluster #12(w522) -> ("定时配置-累积分段.间隔"=w537:u8)
                n102 = Select(t=w535, s=w536, f=w534) -> (s? t:f=w533:bool)
                n103 = case shown="假" w533 {
                  tunnel: w545 -> [w552 w554]
                  tunnel: w544 -> [w551 _]
                  tunnel: w543 -> [w550 _]
                  tunnel: w542 -> [w549 w555]
                  tunnel: [w548 w555] -> w541
                  tunnel: [w547 w554] -> w540
                  tunnel: w539 -> [_ w553]
                  tunnel: [w546 w553] -> w538
                  tunnel: w537 -> [w546 _]
                  frame False {
                    # "没找到, 则写入默认值"
                    n104 = call-poly <vilib>:"Write Key.vi"("section"=w551, "error in (no error)"=w549, "value"=w546, "key"=w550, "refnum"=w552) -> ("error out"=w548:errorcluster, "refnum out"=w547:T10)  [unwired: 4 in, 1 out]
                  }
                  frame True {
                    # "找到则加载"
                  }
                }
                n105 = in-place-cluster #12("定时配置-累积分段.间隔"=w538) -> (w521:T1)
              }
            }
            frame "目标时刻-字符串" {
              n106 = call-poly <vilib>:"Read Key.vi"("section"=w566, "error in (no error)"=w563, "key"=w565, "refnum"=w569) -> ("error out"=w564:errorcluster, "value"=w560:string, "found?"=w568:bool, "refnum out"=w567:T10)  [unwired: 4 in]
              n107 = in-place {
                in-place-border: w568 -> [w571]
                in-place-border: w567 -> [w582]
                in-place-border: w566 -> [w581]
                in-place-border: w565 -> [w580]
                in-place-border: w564 -> [w579]
                in-place-border: [w578] -> w562
                in-place-border: [w577] -> w561
                in-place-border: w560 -> [w576]
                in-place-border: w557 -> [w573]
                in-place-border: w556 -> [w572]
                n108 = in-place-cluster #13(w559) -> ("定时配置-累积分段.目标时刻"=w574:timestamp)
                n109 = Select(t=w573, s=w572, f=w571) -> (s? t:f=w570:bool)
                n110 = case shown="真" w570 {
                  tunnel: w582 -> [w590 w594]
                  tunnel: w581 -> [w589 _]
                  tunnel: w580 -> [w588 _]
                  tunnel: w579 -> [w587 w595]
                  tunnel: [w586 w595] -> w578
                  tunnel: [w585 w594] -> w577
                  tunnel: w576 -> [_ w593]
                  tunnel: [w583 w591] -> w575
                  tunnel: w574 -> [w583 w592]
                  frame False {
                    # "没找到, \n则写入默认值"
                    n111 = Type Cast(x=w583) -> (*(type *) &x=w584:string)  [unwired: 1 in]
                    n112 = call-poly <vilib>:"Write Key.vi"("section"=w589, "error in (no error)"=w587, "value"=w584, "key"=w588, "refnum"=w590) -> ("error out"=w586:errorcluster, "refnum out"=w585:T10)  [unwired: 4 in, 1 out]
                  }
                  frame True {
                    # "找到则加载"
                    n113 = Type Cast(type=w592, x=w593) -> (*(type *) &x=w591:timestamp)
                  }
                }
                n114 = in-place-cluster #13("定时配置-累积分段.目标时刻"=w575) -> (w558:T1)
              }
            }
          }
        }
      }
      frame "自动导出定时" {
        # "自动导出定时段"
        n115 = property on="键-导出定时配置段" class="Enum (严格)"() -> ("Strings []"=w599:string[])  [unwired: 2 in, 2 out]
        n116 = for {
          tunnel: w599 -> [w616] mode=indexing
          tunnel: w605 -> [w612]
          shift-right: [w611] -> w598
          shift-left: w604 -> [w617]
          tunnel: "键-导出定时配置段" -> [w618]
          shift-right: [w610] -> w601
          shift-left: w606 -> [w615]
          shift-right: [w609] -> w602
          shift-left: w603 -> [w614]
          tunnel: w597 -> [w608]
          tunnel: w596 -> [w607]
          i -> [w619]
          # "存在则读取, 不存在则写入默认值"
          n117 = call "Number To Enum.vim"("number"=w619, "enum type"=w618) -> ("number as enum"=w613:T4)
          n118 = case shown="\"定时模式-u32\"" w613 {
            tunnel: w615 -> [w633 w670 w707 w744 w784]
            tunnel: w612 -> [w630 w667 w704 w741 w781]
            tunnel: w616 -> [w629 w666 w703 w740 w780]
            tunnel: w617 -> [w623 w660 w697 w734 w774]
            tunnel: w614 -> [w627 w664 w701 w738 w778]
            tunnel: [w626 w663 w700 w737 w777] -> w609
            tunnel: [w625 w662 w699 w736 w776] -> w610
            tunnel: [w622 w659 w696 w733 w773] -> w611
            tunnel: w608 -> [w621 w658 w695 w732 w772]
            tunnel: w607 -> [w620 w657 w694 w731 w771]
            frame "定时模式-u32" {
              n119 = call-poly <vilib>:"Read Key.vi"("section"=w630, "error in (no error)"=w627, "key"=w629, "refnum"=w633) -> ("error out"=w628:errorcluster, "value"=w624:u32, "found?"=w632:bool, "refnum out"=w631:T10)  [unwired: 4 in]
              n120 = in-place {
                in-place-border: w632 -> [w635]
                in-place-border: w631 -> [w646]
                in-place-border: w630 -> [w645]
                in-place-border: w629 -> [w644]
                in-place-border: w628 -> [w643]
                in-place-border: [w642] -> w626
                in-place-border: [w641] -> w625
                in-place-border: w624 -> [w640]
                in-place-border: w621 -> [w637]
                in-place-border: w620 -> [w636]
                n121 = in-place-cluster #14(w623) -> ("定时配置-自动导出.定时配置-自动导出.定时模式"=w638:enum16{"绝对时间", "相对时间"})
                n122 = Select(t=w636, s=w637, f=w635) -> (s? t:f=w634:bool)
                n123 = case shown="真" w634 {
                  tunnel: w646 -> [w653 w655]
                  tunnel: w645 -> [w652 _]
                  tunnel: w644 -> [w651 _]
                  tunnel: w643 -> [w650 w656]
                  tunnel: [w649 w656] -> w642
                  tunnel: [w648 w655] -> w641
                  tunnel: w640 -> [_ w654]
                  tunnel: [w647 w654] -> w639
                  tunnel: w638 -> [w647 _]
                  frame False {
                    # "没找到, 则写入默认值"
                    n124 = call-poly <vilib>:"Write Key.vi"("section"=w652, "error in (no error)"=w650, "value"=w647, "key"=w651, "refnum"=w653) -> ("error out"=w649:errorcluster, "refnum out"=w648:T10)  [unwired: 4 in, 1 out]
                  }
                  frame True {
                    # "找到则加载"
                  }
                }
                n125 = in-place-cluster #14("定时配置-自动导出.定时配置-自动导出.定时模式"=w639) -> (w622:T1)
              }
            }
            frame "单位-u32" {
              n126 = call-poly <vilib>:"Read Key.vi"("section"=w667, "error in (no error)"=w664, "key"=w666, "refnum"=w670) -> ("error out"=w665:errorcluster, "value"=w661:u32, "found?"=w669:bool, "refnum out"=w668:T10)  [unwired: 4 in]
              n127 = in-place {
                in-place-border: w669 -> [w672]
                in-place-border: w668 -> [w683]
                in-place-border: w667 -> [w682]
                in-place-border: w666 -> [w681]
                in-place-border: w665 -> [w680]
                in-place-border: [w679] -> w663
                in-place-border: [w678] -> w662
                in-place-border: w661 -> [w677]
                in-place-border: w658 -> [w674]
                in-place-border: w657 -> [w673]
                n128 = in-place-cluster #15(w660) -> ("定时配置-自动导出.定时配置-自动导出.单位"=w675:enum16{"年", "月", "日", "时", "分"})
                n129 = Select(t=w673, s=w674, f=w672) -> (s? t:f=w671:bool)
                n130 = case shown="真" w671 {
                  tunnel: w683 -> [w690 w692]
                  tunnel: w682 -> [w689 _]
                  tunnel: w681 -> [w688 _]
                  tunnel: w680 -> [w687 w693]
                  tunnel: [w686 w693] -> w679
                  tunnel: [w685 w692] -> w678
                  tunnel: w677 -> [_ w691]
                  tunnel: [w684 w691] -> w676
                  tunnel: w675 -> [w684 _]
                  frame False {
                    # "没找到, 则写入默认值"
                    n131 = call-poly <vilib>:"Write Key.vi"("section"=w689, "error in (no error)"=w687, "value"=w684, "key"=w688, "refnum"=w690) -> ("error out"=w686:errorcluster, "refnum out"=w685:T10)  [unwired: 4 in, 1 out]
                  }
                  frame True {
                    # "找到则加载"
                  }
                }
                n132 = in-place-cluster #15("定时配置-自动导出.定时配置-自动导出.单位"=w676) -> (w659:T1)
              }
            }
            frame "间隔-u32" {
              n133 = call-poly <vilib>:"Read Key.vi"("section"=w704, "error in (no error)"=w701, "key"=w703, "refnum"=w707) -> ("error out"=w702:errorcluster, "value"=w698:u32, "found?"=w706:bool, "refnum out"=w705:T10)  [unwired: 4 in]
              n134 = in-place {
                in-place-border: w706 -> [w709]
                in-place-border: w705 -> [w720]
                in-place-border: w704 -> [w719]
                in-place-border: w703 -> [w718]
                in-place-border: w702 -> [w717]
                in-place-border: [w716] -> w700
                in-place-border: [w715] -> w699
                in-place-border: w698 -> [w714]
                in-place-border: w695 -> [w711]
                in-place-border: w694 -> [w710]
                n135 = in-place-cluster #16(w697) -> ("定时配置-自动导出.定时配置-自动导出.间隔"=w712:u8)
                n136 = Select(t=w710, s=w711, f=w709) -> (s? t:f=w708:bool)
                n137 = case shown="假" w708 {
                  tunnel: w720 -> [w727 w729]
                  tunnel: w719 -> [w726 _]
                  tunnel: w718 -> [w725 _]
                  tunnel: w717 -> [w724 w730]
                  tunnel: [w723 w730] -> w716
                  tunnel: [w722 w729] -> w715
                  tunnel: w714 -> [_ w728]
                  tunnel: [w721 w728] -> w713
                  tunnel: w712 -> [w721 _]
                  frame False {
                    # "没找到, 则写入默认值"
                    n138 = call-poly <vilib>:"Write Key.vi"("section"=w726, "error in (no error)"=w724, "value"=w721, "key"=w725, "refnum"=w727) -> ("error out"=w723:errorcluster, "refnum out"=w722:T10)  [unwired: 4 in, 1 out]
                  }
                  frame True {
                    # "找到则加载"
                  }
                }
                n139 = in-place-cluster #16("定时配置-自动导出.定时配置-自动导出.间隔"=w713) -> (w696:T1)
              }
            }
            frame "目标时刻-字符串" {
              n140 = call-poly <vilib>:"Read Key.vi"("section"=w741, "error in (no error)"=w738, "key"=w740, "refnum"=w744) -> ("error out"=w739:errorcluster, "value"=w735:string, "found?"=w743:bool, "refnum out"=w742:T10)  [unwired: 4 in]
              n141 = in-place {
                in-place-border: w743 -> [w746]
                in-place-border: w742 -> [w757]
                in-place-border: w741 -> [w756]
                in-place-border: w740 -> [w755]
                in-place-border: w739 -> [w754]
                in-place-border: [w753] -> w737
                in-place-border: [w752] -> w736
                in-place-border: w735 -> [w751]
                in-place-border: w732 -> [w748]
                in-place-border: w731 -> [w747]
                n142 = in-place-cluster #17(w734) -> ("定时配置-自动导出.定时配置-自动导出.目标时刻"=w749:timestamp)
                n143 = Select(t=w747, s=w748, f=w746) -> (s? t:f=w745:bool)
                n144 = case shown="真" w745 {
                  tunnel: w757 -> [w765 w769]
                  tunnel: w756 -> [w764 _]
                  tunnel: w755 -> [w763 _]
                  tunnel: w754 -> [w762 w770]
                  tunnel: [w761 w770] -> w753
                  tunnel: [w760 w769] -> w752
                  tunnel: w751 -> [_ w768]
                  tunnel: [w758 w766] -> w750
                  tunnel: w749 -> [w758 w767]
                  frame False {
                    # "没找到, \n则写入默认值"
                    n145 = Type Cast(x=w758) -> (*(type *) &x=w759:string)  [unwired: 1 in]
                    n146 = call-poly <vilib>:"Write Key.vi"("section"=w764, "error in (no error)"=w762, "value"=w759, "key"=w763, "refnum"=w765) -> ("error out"=w761:errorcluster, "refnum out"=w760:T10)  [unwired: 4 in, 1 out]
                  }
                  frame True {
                    # "找到则加载"
                    n147 = Type Cast(type=w767, x=w768) -> (*(type *) &x=w766:timestamp)
                  }
                }
                n148 = in-place-cluster #17("定时配置-自动导出.定时配置-自动导出.目标时刻"=w750) -> (w733:T1)
              }
            }
            frame "分别导出-布尔" {
              n149 = call-poly <vilib>:"Read Key.vi"("section"=w781, "error in (no error)"=w778, "key"=w780, "refnum"=w784) -> ("error out"=w779:errorcluster, "value"=w775:bool, "found?"=w783:bool, "refnum out"=w782:T10)  [unwired: 4 in]
              n150 = in-place {
                in-place-border: w783 -> [w786]
                in-place-border: w782 -> [w797]
                in-place-border: w781 -> [w796]
                in-place-border: w780 -> [w795]
                in-place-border: w779 -> [w794]
                in-place-border: [w793] -> w777
                in-place-border: [w792] -> w776
                in-place-border: w775 -> [w791]
                in-place-border: w772 -> [w788]
                in-place-border: w771 -> [w787]
                n151 = in-place-cluster #18(w774) -> ("定时配置-自动导出.分别导出?"=w789:bool)
                n152 = Select(t=w787, s=w788, f=w786) -> (s? t:f=w785:bool)
                n153 = case shown="假" w785 {
                  tunnel: w797 -> [w804 w806]
                  tunnel: w796 -> [w803 _]
                  tunnel: w795 -> [w802 _]
                  tunnel: w794 -> [w801 w807]
                  tunnel: [w800 w807] -> w793
                  tunnel: [w799 w806] -> w792
                  tunnel: w791 -> [_ w805]
                  tunnel: [w798 w805] -> w790
                  tunnel: w789 -> [w798 _]
                  frame False {
                    # "没找到, 则写入默认值"
                    n154 = call-poly <vilib>:"Write Key.vi"("section"=w803, "error in (no error)"=w801, "value"=w798, "key"=w802, "refnum"=w804) -> ("error out"=w800:errorcluster, "refnum out"=w799:T10)  [unwired: 4 in, 1 out]
                  }
                  frame True {
                    # "找到则加载"
                  }
                }
                n155 = in-place-cluster #18("定时配置-自动导出.分别导出?"=w790) -> (w773:T1)
              }
            }
          }
        }
      }
    }
  }
  "配置文件 o" <- w22
  n156 = call <vilib>:"Close Config Data.vi"("error in (no error)"=w20, "refnum"=w19) -> ("error out"=→"error out":errorcluster)  [unwired: 8 in, 1 out]
